vi "test Action Update Heater State-Disable Heater.vi"() -> ()   [LabVIEW 2018, in "AllComponentTestes.lvclass"]
uses:
  AllComponentTestes.lvclass
  C:/Program Files/National Instruments/LabVIEW 2018/vi.lib/addons/_JKI Toolkits/VI Tester/TestCase.llb/TestCase.lvclass
  <vilib>/addons/_JKI Toolkits/VI Tester/TestCase.llb/TestCase.lvclass
  Libraries/Thermal Chamber Controller_DQMH/Thermal Chamber Controller_DQMH.lvlib
panel:
  out "TestCase out":refnum<class "TestCase.lvclass">
  in  "TestCase in":refnum<class "AllComponentTestes.lvclass">
  out "error out":errorcluster
  in  "error in (no error)":errorcluster
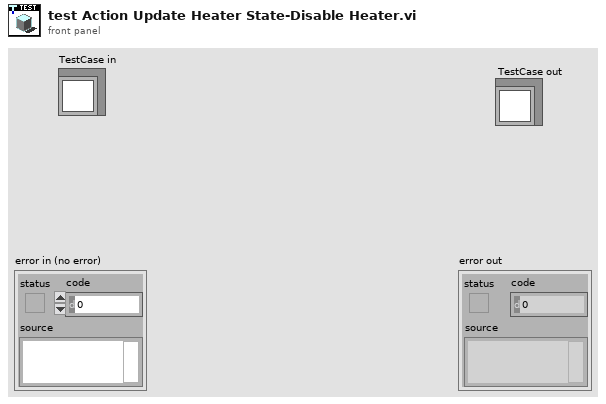
[diagram p1: front panel]
types:
  T1 = typedef "Thermal Chamber Controller_DQMH.lvlib/Heater State--enum.ctl" = enum16{"Heater Enabled", "Heater Disabled"}
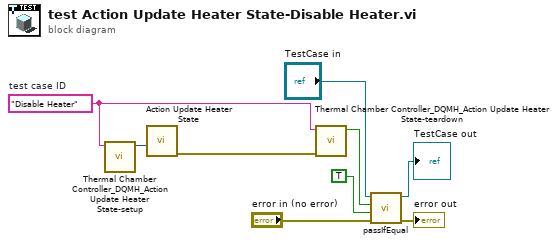
[diagram p0: block diagram]
diagram:
  w2 = "Disable Heater"  # test case ID
  n1 = call "Thermal Chamber Controller_DQMH_Action Update Heater State-setup.vi"("test case ID"=w2) -> ("Heater State"=w3:T1)  [unwired: 10 in]
  n2 = call "Action Update Heater State.vi"("Heater State"=w3) -> ("error out"=w4:errorcluster)  [unwired: 10 in]
  n3 = call "Thermal Chamber Controller_DQMH_Action Update Heater State-teardown.vi"("error in (no error)"=w4, "test case ID"=w2) -> ("result"=w1:bool)  [unwired: 9 in]
  n4 = call-dynamic "passIfEqual.vi"("error in (no error)"="error in (no error)", "y"=TRUE, "x"=w1, "TestCase in"="TestCase in") -> ("error out"=→"error out":errorcluster, "TestCase out"=→"TestCase out":refnum<class "AllComponentTestes.lvclass">)  [unwired: 6 in]
